vi "CompareVIs.vi"() -> ()   [LabVIEW 2022 SP3]
panel:
  out "error out":errorcluster
  out "Same?":bool
  in  "Result JSON Path":path
  in  "ours":path
  in  "Theirs":path
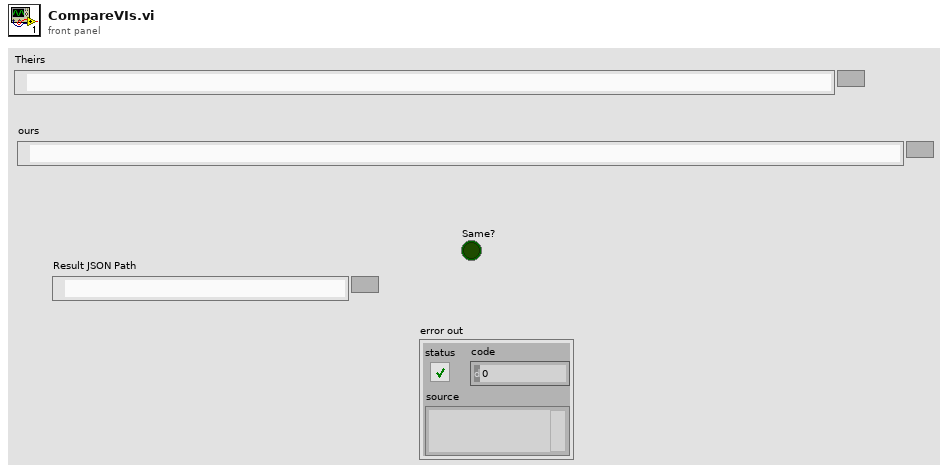
[diagram p1: front panel]
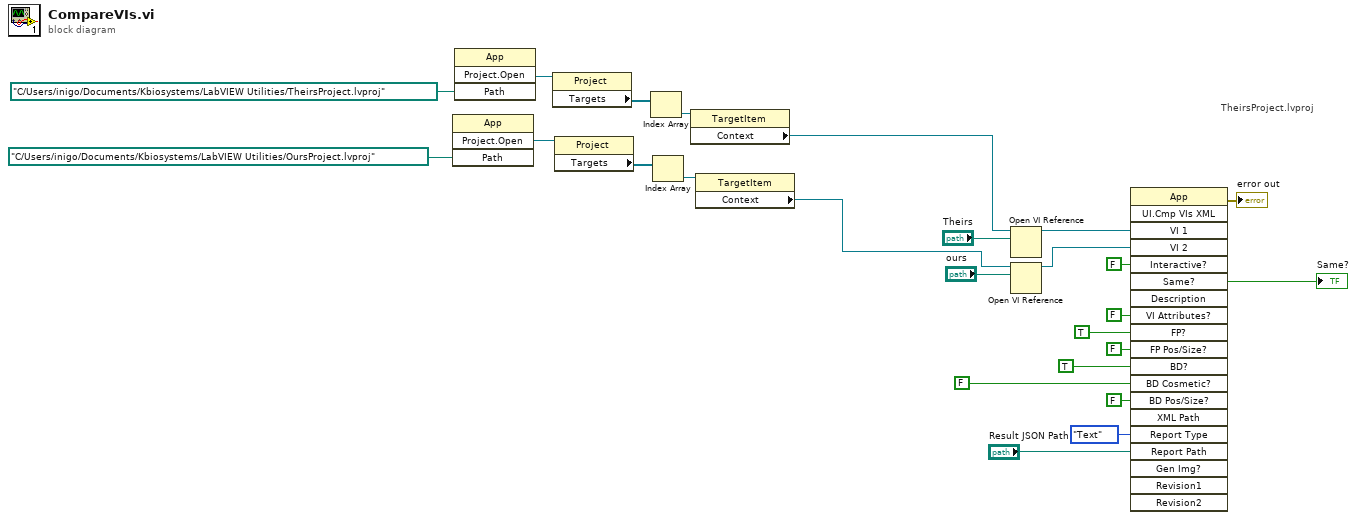
[diagram p0: block diagram]
diagram:
  # "TheirsProject.lvproj"
  n1 = invoke class="App" method="Project.Open"("Path"=path "C:/Users/inigo/Documents/Kbiosystems/LabVIEW Utilities/OursProject.lvproj") -> ("Project:Open"=w11:refnum<vi>)  [unwired: 3 in, 3 out]
  n2 = invoke class="App" method="Project.Open"("Path"=path "C:/Users/inigo/Documents/Kbiosystems/LabVIEW Utilities/TheirsProject.lvproj") -> ("Project:Open"=w14:refnum<vi>)  [unwired: 3 in, 3 out]
  n3 = property class="Project"(reference=w14) -> ("Targets"=w13:refnum<vi>[])  [unwired: 1 in, 2 out]
  n4 = property class="Project"(reference=w11) -> ("Targets"=w12:refnum<vi>[])  [unwired: 1 in, 2 out]
  n5 = Index Array(array=w13) -> (element=w10:refnum<vi>)  [unwired: 1 in]
  n6 = Index Array(array=w12) -> (element=w9:refnum<vi>)  [unwired: 1 in]
  n7 = property class="TargetItem"(reference=w10) -> ("Context"=w8:refnum<vi>)  [unwired: 1 in, 2 out]
  n8 = property class="TargetItem"(reference=w9) -> ("Context"=w7:refnum<vi>)  [unwired: 1 in, 2 out]
  n9 = Open VI Reference(application reference (local)=w8, vi path="Theirs") -> (vi reference=w24:refnum<vi>)  [unwired: 4 in, 1 out]
  n10 = Open VI Reference(application reference (local)=w7, vi path="ours") -> (vi reference=w22:refnum<vi>)  [unwired: 4 in, 1 out]
  n11 = invoke class="App" method="UI.Cmp VIs XML"("VI 1"=w24, "VI 2"=w22, "Interactive?"=FALSE, "VI Attributes?"=FALSE, "FP?"=TRUE, "FP Pos/Size?"=FALSE, "BD?"=TRUE, "BD Cosmetic?"=FALSE, "BD Pos/Size?"=FALSE, "Report Type"=enum32{"None", "Webpage", "Text", "MS Word"}."Text", "Report Path"="Result JSON Path") -> (error out=→"error out":errorcluster, "Same?"=→"Same?":bool)  [unwired: 9 in, 18 out]
